vi "TargetAngle.vi"() -> ()   [LabVIEW 2013]
panel:
  out "XY Graph":cluster{dbl[], dbl[]}(graph)
  in  "Heading Angle":dbl(knob) scale=-2.0..2.0
  in  "Target Angle":dbl(knob) scale=-2.0..2.0
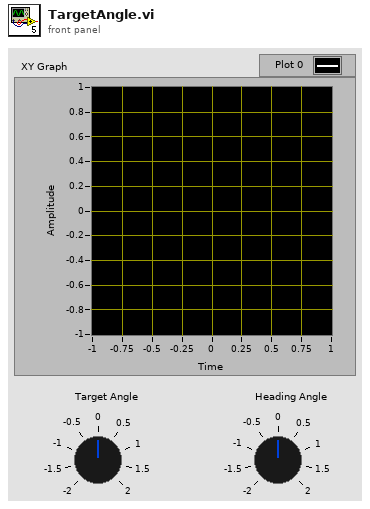
[diagram p1: front panel]
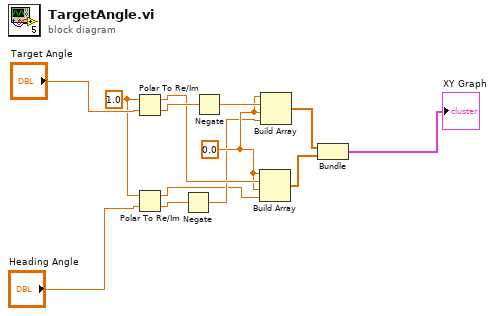
[diagram p0: block diagram]
diagram:
  w3 = 0.0 ("element")
  w11 = 1.0 ("r")
  n1 = Polar To Re/Im(2:"Target Angle", 3:w11) -> (0:w9:dbl, 1:w4:dbl)
  n2 = Polar To Re/Im(2:"Heading Angle", 3:w11) -> (0:w10:dbl, 1:w1:dbl)
  n3 = Negate(x=w10) -> (-x=w2:dbl)
  n4 = Negate(x=w9) -> (-x=w5:dbl)
  n5 = Build Array(w3, w4, w3, w1) -> (w8:dbl[])
  n6 = Build Array(w3, w5, w3, w2) -> (w7:dbl[])
  n7 = Bundle(w7, w8) -> (→"XY Graph":cluster{dbl[], dbl[]})  [unwired: 1 in]
